vi "Dashboard Update.vi"   [LabVIEW 2016]
uses:
  <vilib>/Rock Robotics/Network Tables/NT Read Boolean.vi
  <vilib>/Rock Robotics/Network Tables/NT Read Number.vi
  Robot Values.vi
  <vilib>/Rock Robotics/Network Tables/NT Write Number.vi
  <vilib>/Rock Robotics/Network Tables/NT Write Boolean.vi
  <vilib>/Rock Robotics/Network Tables/NT Write String.vi
  Vision Global.vi
types:
  T1 = typedef "Robot Values.ctl" = cluster{"Robot Drive":cluster{"Left Motor Power":dbl, "Right Motor Power":dbl, "Left Encoder Value":dbl, "Right Encoder Value":dbl, "High Gear?":bool, "PTO?":bool}, "Sensors":cluster{"Gyro Angle":u16, "Recalibrate Gyro":bool, "Reset Gyro":bool, "Ultrasonic":dbl}, "Shooter":cluster{"Prep Wheels":bool, "Shoot":bool, "Left Shooter Wheel Speed":dbl, "Wheels Moving":bool, "Shooter Prepped":bool, "Shooter RPS SP":dbl, "Shooting?":bool, "Left Shooter Wheel Power":dbl, "Right Shooter Wheel Power":dbl, "Acquisition Conveyor Power":dbl, "Hopper Beater Bar Power":dbl, "Filtered Left Shooter Speed":dbl, "Acquisition Motor Power":dbl, "Joystick Add":dbl, "D-Pad Add":dbl, "Shooter Use PID?":bool}, "Robot States":cluster{"Drive mode":string, "Alliance":T2, "Position":T3}, "Gear":cluster{"Ejection Active":bool}}
  T2 = typedef "WPI_DriverStationAllianceInfo.ctl" = enum16{"Red", "Blue", "Invalid"}
  T3 = typedef "WPI_DriverStationPositionInfo.ctl" = enum16{"1", "2", "3"}
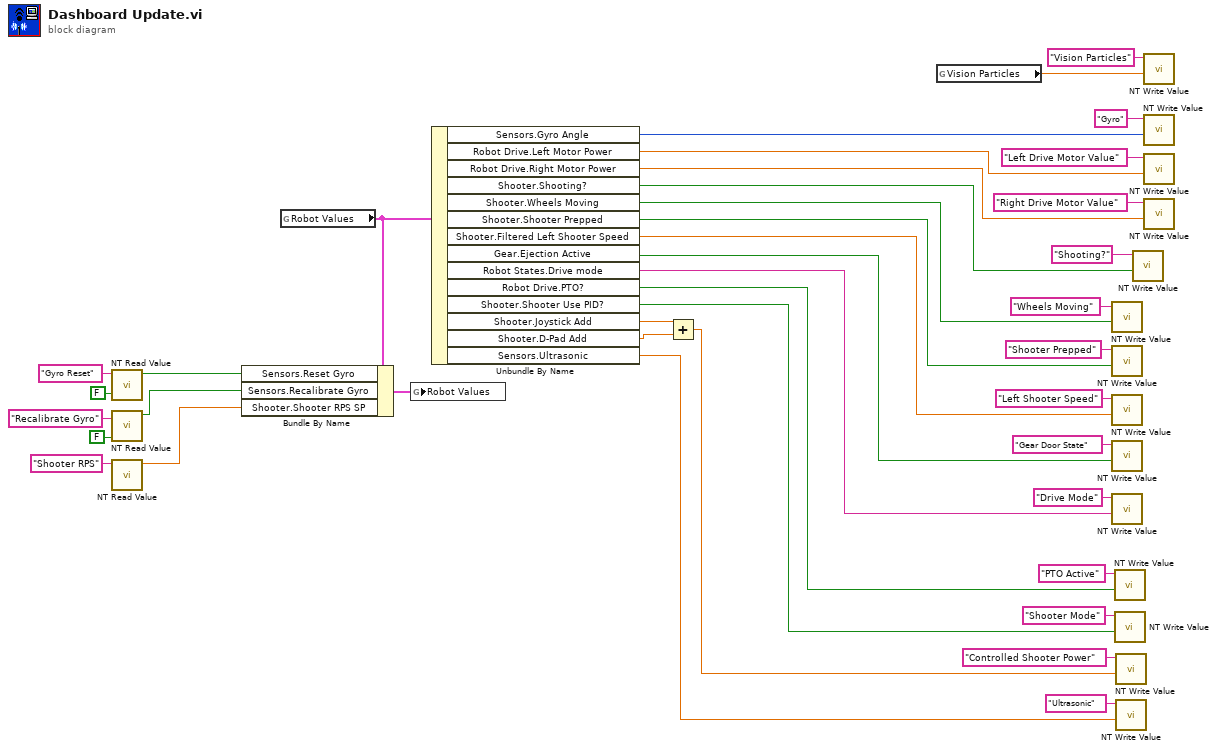
[diagram p0: block diagram]
diagram:
  n1 = call-poly <vilib>:"NT Read Value.vi"("Default Value"=FALSE, "Name"="Gyro Reset") -> ("Boolean"=w31:bool)  [unwired: 8 in, 1 out]
  n2 = call-poly <vilib>:"NT Read Value.vi"("Default Value"=FALSE, "Name"="Recalibrate Gyro") -> ("Boolean"=w27:bool)  [unwired: 8 in, 1 out]
  n3 = call-poly <vilib>:"NT Read Value.vi"("Name"="Shooter RPS") -> ("Numeric"=w17:dbl)  [unwired: 9 in, 1 out]
  n4 = global read "Robot Values.vi" "Robot Values"() -> (w11:T1)
  n5 = Bundle By Name(cluster=w11, "Sensors.Reset Gyro"=w31, "Sensors.Recalibrate Gyro"=w27, "Shooter.Shooter RPS SP"=w17) -> (w32:T1)
  n6 = global write "Robot Values.vi" "Robot Values"(w32) -> ()
  n7 = Unbundle By Name(w11) -> ("Sensors.Gyro Angle"=w40:u16, "Robot Drive.Left Motor Power"=w38:dbl, "Robot Drive.Right Motor Power"=w35:dbl, "Shooter.Shooting?"=w14:bool, "Shooter.Wheels Moving"=w34:bool, "Shooter.Shooter Prepped"=w19:bool, "Shooter.Filtered Left Shooter Speed"=w21:dbl, "Gear.Ejection Active"=w22:bool, "Robot States.Drive mode"=w23:string, "Robot Drive.PTO?"=w12:bool, "Shooter.Shooter Use PID?"=w10:bool, "Shooter.Joystick Add"=w4:dbl, "Shooter.D-Pad Add"=w3:dbl, "Sensors.Ultrasonic"=w1:dbl)
  n8 = Add(x=w4, y=w3) -> (x+y=w8:dbl)
  n9 = global read "Vision Global.vi" "Vision Particles"() -> (w6:dbl)
  n10 = call-poly <vilib>:"NT Write Value.vi"("Boolean"=w34, "Name"="Wheels Moving") -> ()  [unwired: 9 in, 1 out]
  n11 = call-poly <vilib>:"NT Write Value.vi"("Boolean"=w19, "Name"="Shooter Prepped") -> ()  [unwired: 9 in, 1 out]
  n12 = call-poly <vilib>:"NT Write Value.vi"("Numeric"=w21, "Name"="Left Shooter Speed") -> ()  [unwired: 9 in, 1 out]
  n13 = call-poly <vilib>:"NT Write Value.vi"("Boolean"=w22, "Name"="Gear Door State") -> ()  [unwired: 9 in, 1 out]
  n14 = call-poly <vilib>:"NT Write Value.vi"("String"=w23, "Name"="Drive Mode") -> ()  [unwired: 9 in, 1 out]
  n15 = call-poly <vilib>:"NT Write Value.vi"("Boolean"=w12, "Name"="PTO Active") -> ()  [unwired: 9 in, 1 out]
  n16 = call-poly <vilib>:"NT Write Value.vi"("Boolean"=w10, "Name"="Shooter Mode") -> ()  [unwired: 9 in, 1 out]
  n17 = call-poly <vilib>:"NT Write Value.vi"("Numeric"=w8, "Name"="Controlled Shooter Power") -> ()  [unwired: 9 in, 1 out]
  n18 = call-poly <vilib>:"NT Write Value.vi"("Numeric"=w1, "Name"="Ultrasonic") -> ()  [unwired: 9 in, 1 out]
  n19 = call-poly <vilib>:"NT Write Value.vi"("Boolean"=w14, "Name"="Shooting?") -> ()  [unwired: 9 in, 1 out]
  n20 = call-poly <vilib>:"NT Write Value.vi"("Numeric"=w6, "Name"="Vision Particles") -> ()  [unwired: 9 in, 1 out]
  n21 = call-poly <vilib>:"NT Write Value.vi"("Numeric"=w40, "Name"="Gyro") -> ()  [unwired: 9 in, 1 out]
  n22 = call-poly <vilib>:"NT Write Value.vi"("Numeric"=w38, "Name"="Left Drive Motor Value") -> ()  [unwired: 9 in, 1 out]
  n23 = call-poly <vilib>:"NT Write Value.vi"("Numeric"=w35, "Name"="Right Drive Motor Value") -> ()  [unwired: 9 in, 1 out]
